vi "ex_CheckAllT0DtEqual.vi"   [LabVIEW 2017]
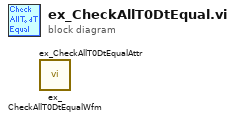
[diagram p0: block diagram]
diagram:
  n1 = call <vilib>:"ex_CheckAllT0DtEqualWfm.vi"() -> ()  [unwired: 1 in, 1 out]
  n2 = call <vilib>:"ex_CheckAllT0DtEqualAttr.vi"() -> ()  [unwired: 1 in, 1 out]
